vi "FunctDataMgr.Function Add RTN Data.vi"(4 "SW Items":T3[](array[typedef]), 6 "Vars":string[][](array[string]), 7 "UUT Props":string[][](array[string]), 8 "Error In":errorcluster, 10 "Meas":T1[](array[typedef]) {"Status" items=["LOG", "PASS", "FAIL", "ERROR"]}, 11 "FunctDataMgr in":refnum<class "FunctDataMgr.lvclass">) -> (3 "FunctDataMgr out":refnum<class "FunctDataMgr.lvclass">)   [LabVIEW 2024, in "FunctDataMgr.lvclass"]
uses:
  FunctDataMgr.lvclass
  Results/Result XML/TestResult.SW Item.ctl
  Results/Result.Measurement Item.ctl
  Results/Result.Measurement and Attribute Item Status.ctl
  FunctDataMgr.lvclass/FunctDataMgr.ctl
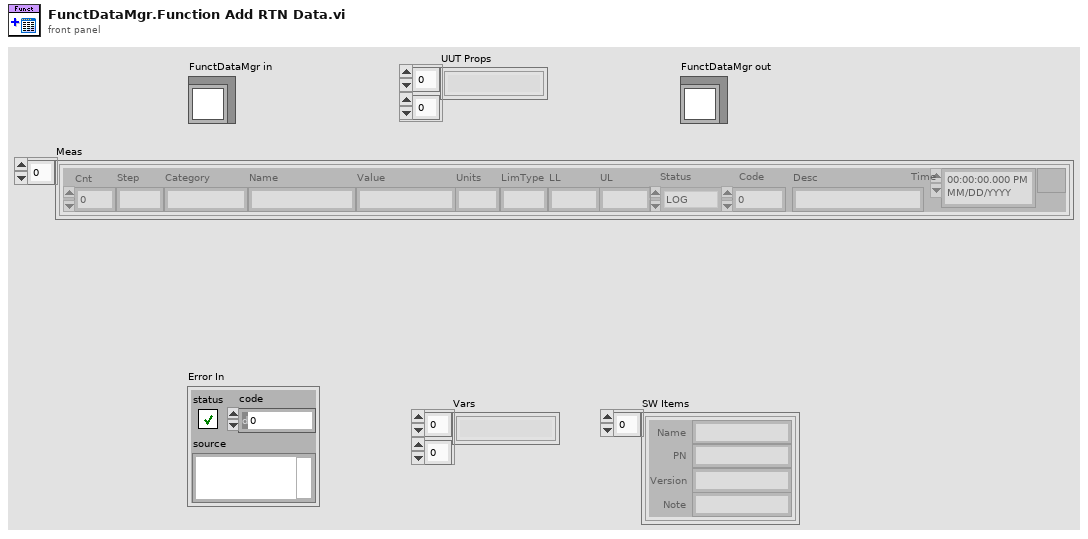
[diagram p1: front panel]
types:
  T1 = typedef "Result.Measurement Item.ctl" = cluster{"Cnt":i32, "Step":string, "Category":string, "Name":string, "Value":string, "Units":string, "LimType":string, "LL":string, "UL":string, "Status":T2, "Code":i32, "Desc":string, "Time":timestamp}
  T2 = typedef "Result.Measurement and Attribute Item Status.ctl" = i32
  T3 = typedef "TestResult.SW Item.ctl" = cluster{"Name":string, "PN":string, "Version":string, "Note":string}
  T4 = typedef "TestExec.Local Result Data.ctl" = cluster{"Attr":T5[], "Num":T6[], "UUT Props":string[][], "Vars":string[][], "SW Items":T3[], "Error":errorcluster, "Step":i32, "FileObjs":T8[], "MeasData":T1[]}
  T5 = typedef "Result.Attribute.ctl" = cluster{"Cnt":i32, "Step":string, "Category":string, "Name":string, "Value":string, "Status":T2, "Code":i32, "Desc":string, "Time":timestamp}
  T6 = typedef "Result.Numeric.ctl" = cluster{"Cnt":i32, "Step":string, "Category":string, "Name":string, "Value":dbl, "Units":string, "LimType":T7, "LL":dbl, "UL":dbl, "Status":T2, "Code":i32, "Desc":string, "Time":timestamp}
  T7 = typedef "Result.Limit Type.ctl" = enum16{"None", "EQ", "NE", "GT", "LT", "GE", "LE", "GTLT", "GELE", "GELT", "GTLE", "LTGT", "LEGE", "LEGT", "LTGE", "Contains", "NotContains"}
  T8 = typedef "Report.Result FileDataObject.ctl" = cluster{"Cnt":i32, "Step":string, "Category":string, "Name":string, "Type":string, "File Name":string, "Time":string, "Path":path}
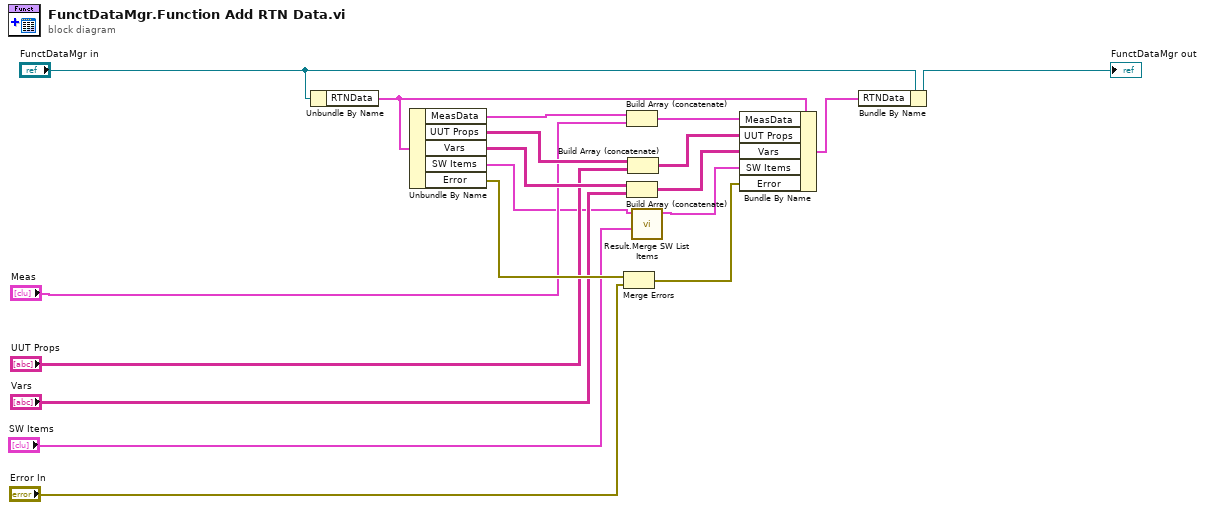
[diagram p0: block diagram]
diagram:
  n1 = Unbundle By Name("FunctDataMgr in") -> ("RTNData"=w16:T4)
  n2 = Unbundle By Name(w16) -> ("MeasData"=w11:T1[], "UUT Props"=w10:string[][], "Vars"=w9:string[][], "SW Items"=w2:T3[], "Error"=w12:errorcluster)
  n3 = Merge Errors(w12, "Error In") -> (w13:errorcluster)
  n4 = Build Array (concatenate)(w11, "Meas") -> (w14:T1[])
  n5 = Build Array (concatenate)(w9, "Vars") -> (w7:string[][])
  n6 = Build Array (concatenate)(w10, "UUT Props") -> (w8:string[][])
  n7 = call "Result.Merge SW List Items.vi"("Old Items"="SW Items", "New Items"=w2) -> ("Merged Items"=w1:T3[])  [unwired: 9 in]
  n8 = Bundle By Name(cluster=w16, "MeasData"=w14, "UUT Props"=w8, "Vars"=w7, "SW Items"=w1, "Error"=w13) -> (w15:T4)
  n9 = Bundle By Name(cluster="FunctDataMgr in", "RTNData"=w15) -> (→"FunctDataMgr out":refnum<class "FunctDataMgr.lvclass">)
